vi "LED Compare.vi"(0 "Actul LED Status":T3={"Deep Rinse"=enum."On", "Wash"=enum."Off", "Rinse"=enum."Off", "Spin"=enum."Off", "Lid Lock"=enum."Off"}, 1 "Expected LED Status":T3={"Deep Rinse"=enum."On", "Wash"=enum."Off", "Rinse"=enum."Off", "Spin"=enum."Off", "Lid Lock"=enum."Off"}, 2 "Care":T1, 11 "Error In":errorcluster) -> (4 "Pass/Fail?":bool, 6 "Report Text":string, 15 "Error Out":errorcluster)   [LabVIEW 2016]
uses:
  type defs/LED Status OOB.ctl
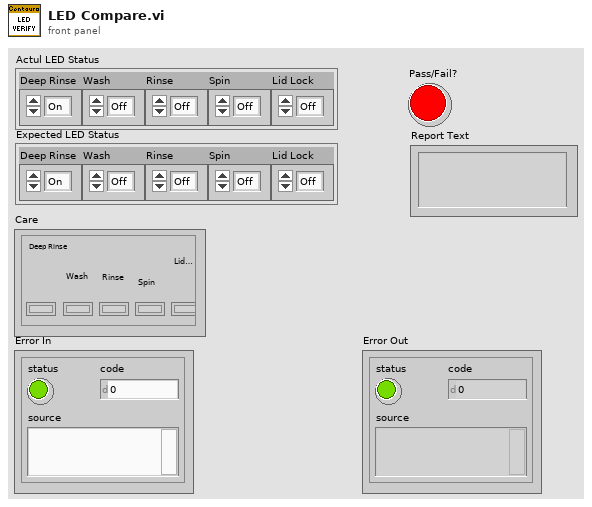
[diagram p1: front panel]
types:
  T1 = cluster{"Deep Rinse":bool, "Wash":bool, "Rinse":bool, "Spin":bool, "Lid Lock":bool}
  T2 = typedef "LED Status OOB.ctl" = enum32{"Off", "On", "Blink"}
  T3 = cluster{"Deep Rinse":T2, "Wash":T2, "Rinse":T2, "Spin":T2, "Lid Lock":T2}
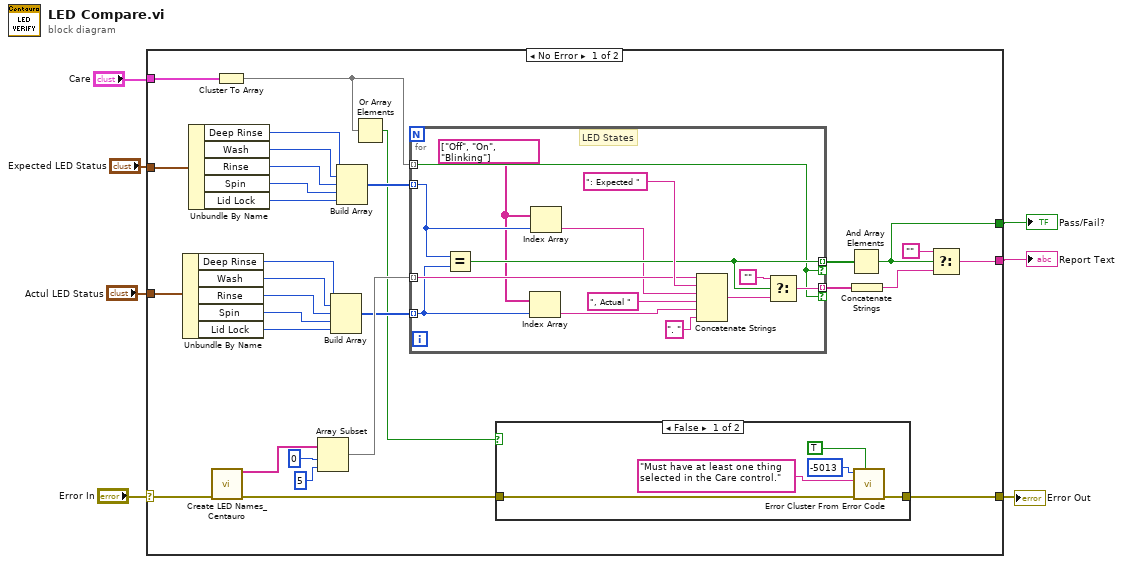
[diagram p0: block diagram]
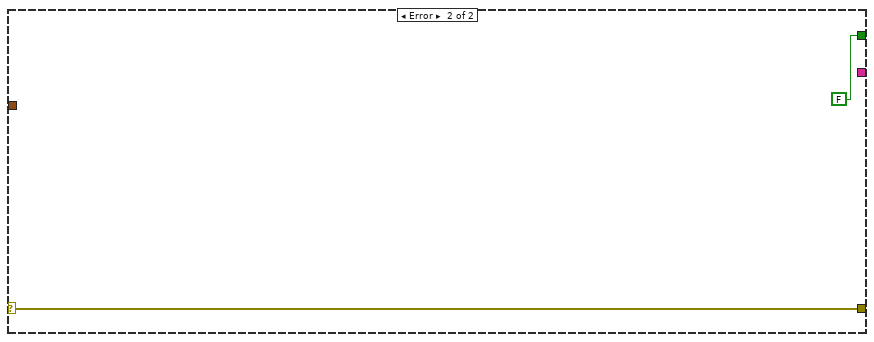
[diagram p3: hidden frame]
diagram:
  n1 = case shown="No Error" "Error In" {
    selector: "Error In" -> [w35 w59]
    tunnel: [w20 w59] -> w1
    tunnel: [w36 _] -> w4
    tunnel: "Care" -> [w34 _]
    tunnel: "Expected LED Status" -> [w17 _]
    tunnel: [w18 FALSE] -> w3
    tunnel: "Actul LED Status" -> [w10 _]
    frame No Error {
      n2 = Unbundle By Name(w10) -> ("Deep Rinse"=w12:T2, "Wash"=w13:T2, "Rinse"=w14:T2, "Spin"=w15:T2, "Lid Lock"=w16:T2)
      n3 = Unbundle By Name(w17) -> ("Deep Rinse"=w24:T2, "Wash"=w23:T2, "Rinse"=w22:T2, "Spin"=w21:T2, "Lid Lock"=w19:T2)
      n4 = call "Create LED Names_Centauro.vi"("Error In"=w35) -> ("Names"=w28:string[], "Error Out"=w33:errorcluster)  [unwired: 13 in]
      n5 = Cluster To Array(cluster=w34) -> (array=w9:bool[])
      n6 = Array Subset(array=w28, index=0, length=5) -> (w29:string[])
      n7 = Build Array(w12, w13, w14, w15, w16) -> (w11:T2[])
      n8 = Build Array(w24, w23, w22, w21, w19) -> (w32:T2[])
      n9 = Or Array Elements(Boolean array=w9) -> (logical OR=w8:bool)
      n10 = for {
        tunnel: w11 -> [w38] mode=indexing
        tunnel: w32 -> [w41] mode=indexing
        tunnel: [w46] -> w27 mode=indexing if=w44
        tunnel: [w45] -> w25 mode=indexing if=w44
        tunnel: w9 -> [w44] mode=indexing
        tunnel: w29 -> [w43] mode=indexing
        w39 = string[] ["Off", "On", "Blinking"]
        # "LED States"
        n11 = Equal?(x=w41, y=w38) -> (x = y?=w45:bool)
        n12 = Index Array(array=w39, index=w38) -> (element=w40:string)
        n13 = Index Array(array=w39, index=w41) -> (element=w42:string)
        n14 = Concatenate Strings(w43, ": Expected " ("string"), w42, ", Actual " ("string"), w40, ". " ("string")) -> (w47:string)
        n15 = Select(t="", s=w45, f=w47) -> (s? t:f=w46:string)
      }
      n16 = case shown="False" w8 {
        tunnel: w33 -> [w56 w57]
        tunnel: [w55 w57] -> w20
        frame False {
          n17 = call <vilib>:"Error Cluster From Error Code.vi"("show call chain? (False)"=TRUE, "error in (no error)"=w56, "error message (\"\")"="Must have at least one thing selected in the Care control." ("error message (\"\")"), "error code (0)"=-5013) -> ("error out"=w55:errorcluster)  [unwired: 5 in]
        }
        frame True {
        }
      }
      n18 = And Array Elements(Boolean array=w25) -> (logical AND=w18:bool)
      n19 = Concatenate Strings(w27) -> (w26:string)
      n20 = Select(t="", s=w18, f=w26) -> (s? t:f=w36:string)
    }
    frame Error {
    }
  }
  "Report Text" <- w4
  "Pass/Fail?" <- w3
  "Error Out" <- w1
